vi "GLOBAL_VAR.vi"() -> ()   [LabVIEW 2018]
panel:
  in  "PB_spinapi_path":path=path "C:/SpinCore/SpinAPI/lib/spinapi64.dll"
  in  "Kz_volt":dbl=0.1 caption="Kz="
  in  "Ky_volt":dbl=1.0 caption="Ky="
  in  "Kx_volt":dbl=1.0 caption="Kx="
  in  "Kz_air":dbl=0.1 caption="Kz="
  in  "Ky_air":dbl=0.016065 caption="Ky="
  in  "Kx_air":dbl=0.01679 caption="Kx="
  in  "Kz_Oil":dbl=0.1 caption="Kz="
  in  "Ky_oil":dbl=0.03104 caption="Ky="
  in  "Kx_oil":dbl=-0.03219 caption="Kx="
  in  "power_factor":dbl=115000.0 format="%#_6e"
  in  "PB_trigger_counter":tag="Dev1/ctr2"
  in  "PB_trigger_in":tag="/Dev1/PFI2"
  in  "COM_MWgenerator":string(combo)="COM4" caption="Generator\nCOM port :"
  in  "MW_generator":enum32{"Hittite", "Rohde & Schwarz"}(radio)=enum."Rohde & Schwarz" caption="Microwave generator :"
  in  "Motors-enable":bool caption="Enable :"
  in  "Z_min_um":dbl caption="Z min mm :" min=0.0 max=10.0
  in  "Z_max_um":dbl=100.0 caption="Z max mm :" min=0.0 max=10.0
  in  "Motor_speed_z":dbl=0.4 caption="Z:" min=0.0 max=25.0 format="%#.3f"
  in  "Motor_speed_xy":dbl=0.4 caption="X, Y:" min=0.0 max=25.0 format="%#.3f"
  in  "Motor_xy_increment":dbl=0.01 caption="Increment [mm]" min=0.0 max=25.0 step=0.001 format="%.3f"
  in  "Motor_z_max":dbl=11.0 caption="Z:" min=0.0 max=25.0 format="%#.3f"
  in  "Motor_y_max":dbl=8.0 caption="Y:" min=0.0 max=25.0 format="%#.3f"
  in  "Motor_x_max":dbl=8.0 caption="X:" min=0.0 max=25.0 format="%#.3f"
  in  "Motor_z_min":dbl caption="Z:" min=0.0 max=25.0 format="%#.3f"
  in  "Motor_y_min":dbl caption="Y:" min=0.0 max=25.0 format="%#.3f"
  in  "Motor_x_min":dbl caption="X:" min=0.0 max=25.0 format="%#.3f"
  in  "COM_Z":string(combo)="COM6" caption="Z:"
  in  "COM_Y":string(combo)="COM5" caption="Y:"
  in  "COM_X":string(combo)="COM7" caption="X:"
  in  "Z_min_v":dbl caption="Z min volts :" min=0.0 max=10.0
  in  "Z_max_v":dbl=10.0 caption="Z max volts :" min=0.0 max=10.0
  in  "XY_min_v":dbl=-10.0 caption="X,Y min volts :" min=-10.0 max=10.0
  in  "XY_max_v":dbl=10.0 caption="X,Y max volts :" min=-10.0 max=10.0
  in  "Kz":dbl=0.1 caption="Kz="
  in  "Ky":dbl=0.042 caption="Ky="
  in  "Kx":dbl=0.042 caption="Kx="
  in  "APD_filter_counter_out":tag="/Dev1/Ctr1InternalOutput"
  in  "APD_filter_counter":tag="Dev1/ctr1"
  in  "APD_counter_clock":tag="/Dev1/100MHzTimebase"
  in  "APD_signal":tag="/Dev1/PFI8"
  in  "APD_counter_trigger_in":tag="/Dev1/PFI0"
  in  "APD_counter_trigger_out":tag="Dev1/port0/line1"
  in  "Gate":tag="Dev1/ctr3"
  in  "Gate input":tag="/Dev1/PFI15"
  in  "APD_counter":tag="Dev1/ctr0"
  in  "X_aoChan":tag="Dev1/ao0"
  in  "Z_aoChan":tag="Dev1/ao2"
  in  "Y_aoChan":tag="Dev1/ao1"
  # "Analog Outputs"
  # "Objective - scale constants"
  # "V/um"
  # "Curent values"
  # "Oil Objectives"
  # "Air objectives"
  # "Direct Voltage"
  # "Vx = Kx * Lx"
  # "Vy = Ky * Ly"
  # "Vz = Kz * Lz"
  # "Last update: begining of 2018"
  # "Galvo mirrors range"
  # "APD counters"
  # "Microware generators"
  # "ctr0"
  # "Piezo positioner range"
  # "ctr3"
  # "PFI15"
  # "Micro positioners (motors)"
  # "PulseBlaster"
  # "port0/line1"
  # "PFI0"
  # "Motors range"
  # "COM channels"
  # "Min."
  # "Max."
  # "PFI8"
  # "[mm]"
  # "APD signal dead time"
  # "Power meter"
  # "Speed [mm/s]"
  # "Step size X,Y"
  # "ctr1"
  # "The value was obtained\nempirically.\nThe instrument gives the\npower in Watts."
  # "Ctr1InternalOutput"
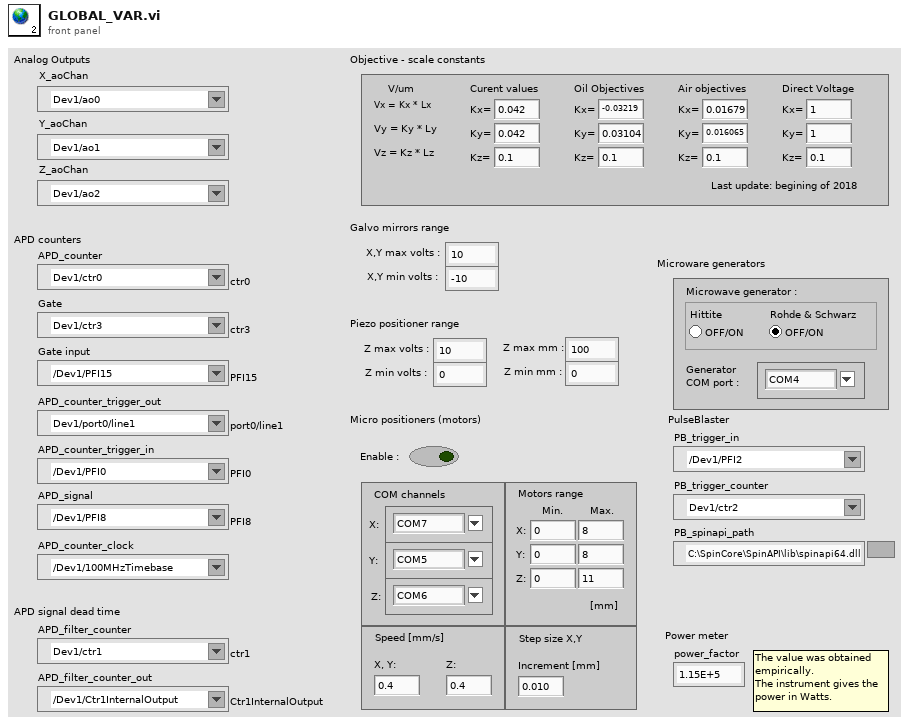
[diagram p1: front panel]
diagram:
